vi "setCatapultMotor.vi"(8 "Ready":bool, 9 "Shooting Time":u32, 10 "Front Pass":bool, 11 "Back Pass":bool) -> (3 "f":dbl)   [LabVIEW 2014]
uses:
  LabVIEW Data/2015 Beta Robot Project/Robot Global Data.vi
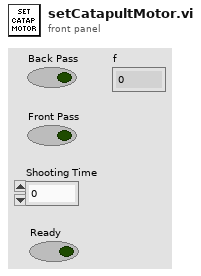
[diagram p1: front panel]
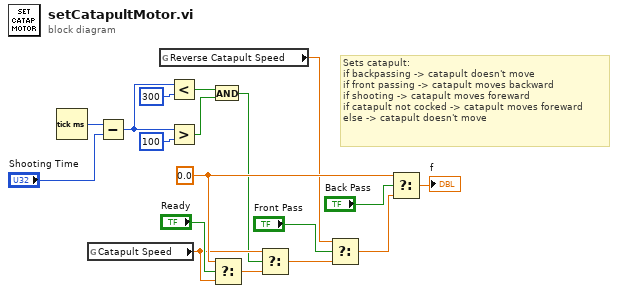
[diagram p0: block diagram]
diagram:
  w11 = 0.0 ("t")
  # "Sets catapult:\nif backpassing -> catapult doesn't move\nif front passing -> catapult moves backward\nif shooting -> catapult moves foreward\nif catapult not cocked -> catapult moves foreward\nelse -> catapult doesn't move"
  n1 = Tick Count (ms)() -> (millisecond timer value=w7:u32)
  n2 = global read "Robot Global Data.vi" "Catapult Speed"() -> (w8:dbl)
  n3 = Subtract(x=w7, y="Shooting Time") -> (x-y=w1:u32)
  n4 = global read "Robot Global Data.vi" "Reverse Catapult Speed"() -> (w9:dbl)
  n5 = Less?(x=w1, y=u32 300) -> (x < y?=w5:bool)
  n6 = Greater?(x=w1, y=u32 100) -> (0:w4:bool)
  n7 = And(x=w5, y=w4) -> (x .and. y?=w3:bool)
  n8 = Select(t=w11, s="Ready", f=w8) -> (s? t:f=w13:dbl)
  n9 = Select(t=w8, s=w3, f=w13) -> (s? t:f=w14:dbl)
  n10 = Select(t=w9, s="Front Pass", f=w14) -> (s? t:f=w17:dbl)
  n11 = Select(t=w11, s="Back Pass", f=w17) -> (s? t:f=→"f":dbl)
